vi "Build Legal Info Sub Section.vi"(8 "error in":errorcluster, 11 "Has DQMH modules":bool) -> (0 "error out":errorcluster, 3 "Lv Proj Document Type:TAF Proj":refnum<class "Sub Section.lvclass">)   [LabVIEW 2021, in "TAF Proj Document Type.lvlib" / "TAF Proj.lvclass"]
uses:
  <vilib>/Wovalab/AntiDoc/Document Type/Add-ons/LabVIEW TAF Project/TAF Proj/TAF Proj.lvclass
  <vilib>/Wovalab/AntiDoc/Sub Section/Sub Section.lvclass
  <vilib>/Wovalab/AsciiDoc for LabVIEW/Paragraph/Paragraph.lvclass
  C:/Program Files (x86)/National Instruments/LabVIEW 2021/vi.lib/Wovalab/AsciiDoc for LabVIEW/Adoc-Bloc/Bloc.lvclass
  <vilib>/Wovalab/AntiDoc/Bloc/Bloc.lvclass
  <vilib>/Wovalab/AntiDoc/Section/Section.lvclass
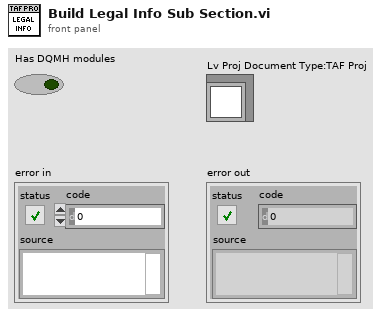
[diagram p1: front panel]
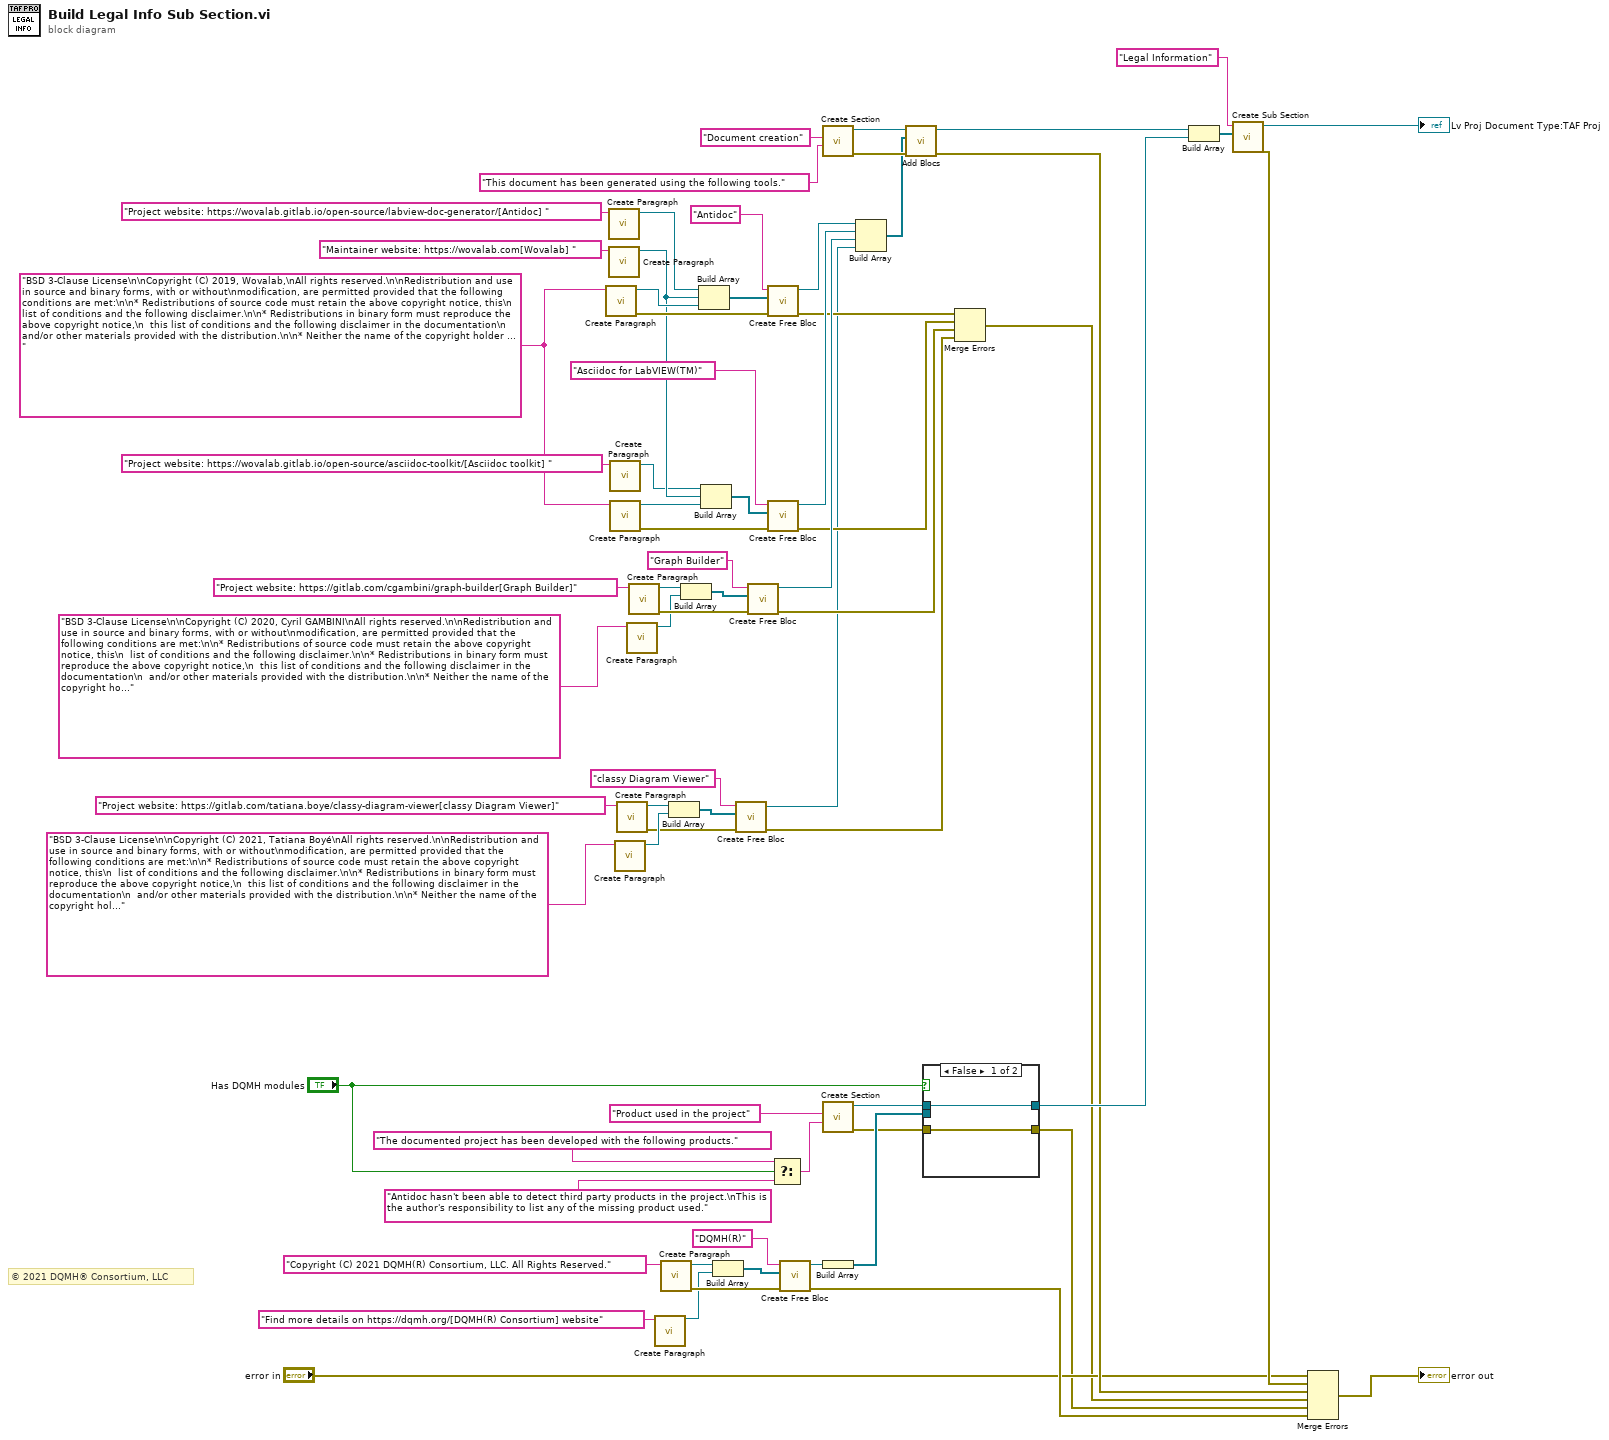
[diagram p0: block diagram]
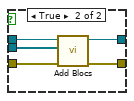
[diagram p2: hidden frame]
diagram:
  w63 = "BSD 3-Clause License\n\nCopyright (C) 2019, Wovalab,\nAll rights reserved.\n\nRedistribution and use in source and binary forms, with or without\nmodification, are permitted provided that the following conditions are met:\n\n* Redistributions of source code must retain the above copyright notice, this\n  list of conditions and the following disclaimer.\n\n* Redistributions in binary form must reproduce the above copyright notice,\n  this list of conditions and the following disclaimer in the documentation\n  and/or other materials provided with the distribution.\n\n* Neither the name of the copyright holder nor the names of its\n  contributors may be used to endorse or promote products derived from\n  this software without specific prior written permission.\n\nTHIS SOFTWARE IS PROVIDED BY THE COPYRIGHT HOLDERS AND CONTRIBUTORS \"AS IS\"\nAND ANY EXPRESS OR IMPLIED WARRANTIES, INCLUDING, BUT NOT LIMITED TO, THE\nIMPLIED WARRANTIES OF MERCHANTABILITY AND FITNESS FOR A PARTICULAR PURPOSE ARE\nDISCLAIMED. IN NO EVENT SHALL THE COPYRIGHT HOLDER OR CONTRIBUTORS BE LIABLE\nFOR ANY DIRECT, INDIRECT, INCIDENTAL, SPECIAL, EXEMPLARY, OR CONSEQUENTIAL\nDAMAGES (INCLUDING, BUT NOT LIMITED TO, PROCUREMENT OF SUBSTITUTE GOODS OR\nSERVICES; LOSS OF USE, DATA, OR PROFITS; OR BUSINESS INTERRUPTION) HOWEVER\nCAUSED AND ON ANY THEORY OF LIABILITY, WHETHER IN CONTRACT, STRICT LIABILITY,\nOR TORT (INCLUDING NEGLIGENCE OR OTHERWISE) ARISING IN ANY WAY OUT OF THE USE\nOF THIS SOFTWARE, EVEN IF ADVISED OF THE POSSIBILITY OF SUCH DAMAGE." ("Content")
  # "© 2021 DQMH® Consortium, LLC"
  n1 = call <vilib>:"Create Paragraph.vi"("Content"=w63) -> ("error out"=w67:errorcluster, "Paragraph out"=w50:refnum<class "Paragraph.lvclass">)  [unwired: 9 in]
  n2 = call <vilib>:"Create Paragraph.vi"("Content"="Project website: https://wovalab.gitlab.io/open-source/labview-doc-generator/[Antidoc] ") -> ("Paragraph out"=w19:refnum<class "Paragraph.lvclass">)  [unwired: 9 in, 1 out]
  n3 = call <vilib>:"Create Paragraph.vi"("Content"="Maintainer website: https://wovalab.com[Wovalab] ") -> ("Paragraph out"=w16:refnum<class "Paragraph.lvclass">)  [unwired: 9 in, 1 out]
  n4 = call <vilib>:"Create Paragraph.vi"("Content"="Project website: https://wovalab.gitlab.io/open-source/asciidoc-toolkit/[Asciidoc toolkit] ") -> ("Paragraph out"=w14:refnum<class "Paragraph.lvclass">)  [unwired: 9 in, 1 out]
  n5 = call <vilib>:"Create Paragraph.vi"("Content"=w63) -> ("error out"=w70:errorcluster, "Paragraph out"=w59:refnum<class "Paragraph.lvclass">)  [unwired: 9 in]
  n6 = call <vilib>:"Create Paragraph.vi"("Content"="BSD 3-Clause License\n\nCopyright (C) 2021, Tatiana Boyé\nAll rights reserved.\n\nRedistribution and use in source and binary forms, with or without\nmodification, are permitted provided that the following conditions are met:\n\n* Redistributions of source code must retain the above copyright notice, this\n  list of conditions and the following disclaimer.\n\n* Redistributions in binary form must reproduce the above copyright notice,\n  this list of conditions and the following disclaimer in the documentation\n  and/or other materials provided with the distribution.\n\n* Neither the name of the copyright holder nor the names of its\n  contributors may be used to endorse or promote products derived from\n  this software without specific prior written permission.\n\nTHIS SOFTWARE IS PROVIDED BY THE COPYRIGHT HOLDERS AND CONTRIBUTORS \"AS IS\"\nAND ANY EXPRESS OR IMPLIED WARRANTIES, INCLUDING, BUT NOT LIMITED TO, THE\nIMPLIED WARRANTIES OF MERCHANTABILITY AND FITNESS FOR A PARTICULAR PURPOSE ARE\nDISCLAIMED. IN NO EVENT SHALL THE COPYRIGHT HOLDER OR CONTRIBUTORS BE LIABLE\nFOR ANY DIRECT, INDIRECT, INCIDENTAL, SPECIAL, EXEMPLARY, OR CONSEQUENTIAL\nDAMAGES (INCLUDING, BUT NOT LIMITED TO, PROCUREMENT OF SUBSTITUTE GOODS OR\nSERVICES; LOSS OF USE, DATA, OR PROFITS; OR BUSINESS INTERRUPTION) HOWEVER\nCAUSED AND ON ANY THEORY OF LIABILITY, WHETHER IN CONTRACT, STRICT LIABILITY,\nOR TORT (INCLUDING NEGLIGENCE OR OTHERWISE) ARISING IN ANY WAY OUT OF THE USE\nOF THIS SOFTWARE, EVEN IF ADVISED OF THE POSSIBILITY OF SUCH DAMAGE.\n") -> ("Paragraph out"=w8:refnum<class "Paragraph.lvclass">)  [unwired: 9 in, 1 out]
  n7 = call <vilib>:"Create Paragraph.vi"("Content"="Project website: https://gitlab.com/tatiana.boye/classy-diagram-viewer[classy Diagram Viewer]") -> ("error out"=w5:errorcluster, "Paragraph out"=w4:refnum<class "Paragraph.lvclass">)  [unwired: 9 in]
  n8 = call <vilib>:"Create Paragraph.vi"("Content"="BSD 3-Clause License\n\nCopyright (C) 2020, Cyril GAMBINI\nAll rights reserved.\n\nRedistribution and use in source and binary forms, with or without\nmodification, are permitted provided that the following conditions are met:\n\n* Redistributions of source code must retain the above copyright notice, this\n  list of conditions and the following disclaimer.\n\n* Redistributions in binary form must reproduce the above copyright notice,\n  this list of conditions and the following disclaimer in the documentation\n  and/or other materials provided with the distribution.\n\n* Neither the name of the copyright holder nor the names of its\n  contributors may be used to endorse or promote products derived from\n  this software without specific prior written permission.\n\nTHIS SOFTWARE IS PROVIDED BY THE COPYRIGHT HOLDERS AND CONTRIBUTORS \"AS IS\"\nAND ANY EXPRESS OR IMPLIED WARRANTIES, INCLUDING, BUT NOT LIMITED TO, THE\nIMPLIED WARRANTIES OF MERCHANTABILITY AND FITNESS FOR A PARTICULAR PURPOSE ARE\nDISCLAIMED. IN NO EVENT SHALL THE COPYRIGHT HOLDER OR CONTRIBUTORS BE LIABLE\nFOR ANY DIRECT, INDIRECT, INCIDENTAL, SPECIAL, EXEMPLARY, OR CONSEQUENTIAL\nDAMAGES (INCLUDING, BUT NOT LIMITED TO, PROCUREMENT OF SUBSTITUTE GOODS OR\nSERVICES; LOSS OF USE, DATA, OR PROFITS; OR BUSINESS INTERRUPTION) HOWEVER\nCAUSED AND ON ANY THEORY OF LIABILITY, WHETHER IN CONTRACT, STRICT LIABILITY,\nOR TORT (INCLUDING NEGLIGENCE OR OTHERWISE) ARISING IN ANY WAY OUT OF THE USE\nOF THIS SOFTWARE, EVEN IF ADVISED OF THE POSSIBILITY OF SUCH DAMAGE.") -> ("Paragraph out"=w11:refnum<class "Paragraph.lvclass">)  [unwired: 9 in, 1 out]
  n9 = call <vilib>:"Create Paragraph.vi"("Content"="Project website: https://gitlab.com/cgambini/graph-builder[Graph Builder]") -> ("error out"=w27:errorcluster, "Paragraph out"=w28:refnum<class "Paragraph.lvclass">)  [unwired: 9 in]
  n10 = call <vilib>:"Create Paragraph.vi"("Content"="Find more details on https://dqmh.org/[DQMH(R) Consortium] website") -> ("Paragraph out"=w12:refnum<class "Paragraph.lvclass">)  [unwired: 9 in, 1 out]
  n11 = call <vilib>:"Create Paragraph.vi"("Content"="Copyright (C) 2021 DQMH(R) Consortium, LLC. All Rights Reserved.") -> ("error out"=w68:errorcluster, "Paragraph out"=w55:refnum<class "Paragraph.lvclass">)  [unwired: 9 in]
  n12 = Build Array(w4, w8) -> (w3:refnum<class "Paragraph.lvclass">[])
  n13 = Build Array(w28, w11) -> (w29:refnum<class "Paragraph.lvclass">[])
  n14 = Build Array(w19, w16, w50) -> (w51:refnum<class "Paragraph.lvclass">[])
  n15 = Build Array(w14, w16, w59) -> (w58:refnum<class "Paragraph.lvclass">[])
  n16 = Build Array(w55, w12) -> (w54:refnum<class "Paragraph.lvclass">[])
  n17 = call <vilib>:"Create Free Bloc.vi"("error in"=w5, "Content"=w3, "Name"="classy Diagram Viewer") -> ("error out"=w1:errorcluster, "Bloc out"=w2:refnum<class "Bloc.lvclass">)  [unwired: 7 in]
  n18 = call <vilib>:"Create Free Bloc.vi"("error in"=w27, "Content"=w29, "Name"="Graph Builder") -> ("error out"=w22:errorcluster, "Bloc out"=w24:refnum<class "Bloc.lvclass">)  [unwired: 7 in]
  n19 = call <vilib>:"Create Free Bloc.vi"("error in"=w67, "Content"=w51, "Name"="Antidoc") -> ("error out"=w21:errorcluster, "Bloc out"=w52:refnum<class "Bloc.lvclass">)  [unwired: 7 in]
  n20 = call <vilib>:"Create Free Bloc.vi"("error in"=w70, "Content"=w58, "Name"="Asciidoc for LabVIEW(TM)") -> ("error out"=w23:errorcluster, "Bloc out"=w61:refnum<class "Bloc.lvclass">)  [unwired: 7 in]
  n21 = Select(t="The documented project has been developed with the following products." ("Description"), s="Has DQMH modules", f="Antidoc hasn't been able to detect third party products in the project.\nThis is the author's responsibility to list any of the missing product used." ("Description")) -> (s? t:f=w33:string)
  n22 = call <vilib>:"Create Free Bloc.vi"("error in"=w68, "Content"=w54, "Name"="DQMH(R)") -> ("error out"=w38:errorcluster, "Bloc out"=w66:refnum<class "Bloc.lvclass">)  [unwired: 7 in]
  n23 = call <vilib>:"Create Section.vi"("Description"="This document has been generated using the following tools.", "Name"="Document creation") -> ("error out"=w69:errorcluster, "Section out"=w48:refnum<class "Section.lvclass">)  [unwired: 8 in]
  n24 = call <vilib>:"Create Section.vi"("Description"=w33, "Name"="Product used in the project") -> ("error out"=w31:errorcluster, "Section out"=w42:refnum<class "Section.lvclass">)  [unwired: 8 in]
  n25 = Build Array(w66) -> (w65:refnum<class "Bloc.lvclass">[])
  n26 = Build Array(w52, w61, w24, w2) -> (w53:refnum<class "Bloc.lvclass">[])
  n27 = call <vilib>:"Add Blocs.vi"("error in (no error)"=w69, "Blocs"=w53, "Section in"=w48) -> ("error out"=w39:errorcluster, "Section out"=w49:refnum<class "Section.lvclass">)  [unwired: 7 in]
  n28 = case shown="False" "Has DQMH modules" {
    tunnel: w65 -> [_ w77]
    tunnel: w42 -> [w72 w76]
    tunnel: [w72 w75] -> w41
    tunnel: w31 -> [w71 w74]
    tunnel: [w71 w73] -> w30
    frame False {
    }
    frame True {
      n29 = call <vilib>:"Add Blocs.vi"("error in (no error)"=w74, "Blocs"=w77, "Section in"=w76) -> ("error out"=w73:errorcluster, "Section out"=w75:refnum<class "Section.lvclass">)  [unwired: 7 in]
    }
  }
  n30 = Merge Errors(w21, w23, w22, w1) -> (w20:errorcluster)
  n31 = Build Array(w49, w41) -> (w46:refnum<class "Section.lvclass">[])
  n32 = call <vilib>:"Create Sub Section.vi"("Sections"=w46, "Name"="Legal Information") -> ("error out"=w40:errorcluster, "Sub Section out"=→"Lv Proj Document Type:TAF Proj":refnum<class "Sub Section.lvclass">)  [unwired: 8 in]
  n33 = Merge Errors("error in", w40, w39, w20, w30, w38) -> (→"error out":errorcluster)
